vi "WPI_CameraBackground Loop.vi"(11 "CameraDevRef":T1) -> ()   [LabVIEW 2015]
doc: "This VI acquires the image buffer from the camera MJPG stream at the configured fps rate. It notifies any waiting VIs and allows them to pick up the latest image. This allows the camera and robot vision loop to run at different rates. The 1011, camera is far more efficient using MJPGs, and generally, this is probably the better choice for the camera loop.\n \nThis software is licensed. Open the labview\\readme\\WPI Robotics Library Open Source License.txt file for more information."
uses:
  <vilib>/Rock Robotics/WPI/Camera/WPI_CameraDevRef.ctl
  <vilib>/Rock Robotics/WPI/Camera/WPI_CameraSettings Operations.ctl
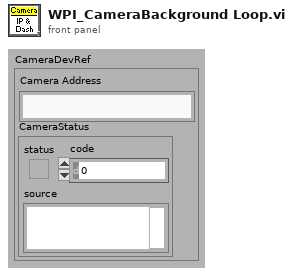
[diagram p1: front panel]
types:
  T1 = typedef "WPI_CameraDevRef.ctl" = cluster{"Camera Address":string, "CameraStatus":errorcluster}
  T2 = typedef "WPI_CameraSettings Operations.ctl" = enum16{"Udate FPS", "Update Compression", "Update Size", "Update White Balance", "Update Brightness", "Update Sharpness", "Update Exposure", "Update Exposure Value", "Update Color Level", "Update Exp Priority", "Update Color Enable", "Update JPG", "Update MJPG", "Read and Clear", "Read", "Init"}
  T3 = typedef "WPI_CameraSettings Control.ctl" = cluster{"FPS":i32, "Compression":i32, "Size":i32, "White Balance":i32, "Brightness":i32, "Sharpness":i32, "Exposure":i32, "Color Level":i32, "Exposure Priority":i32, "Color Enable":i32, "JPG Loop":i32, "MJPG Loop":i32, "Exposure Value":i32}
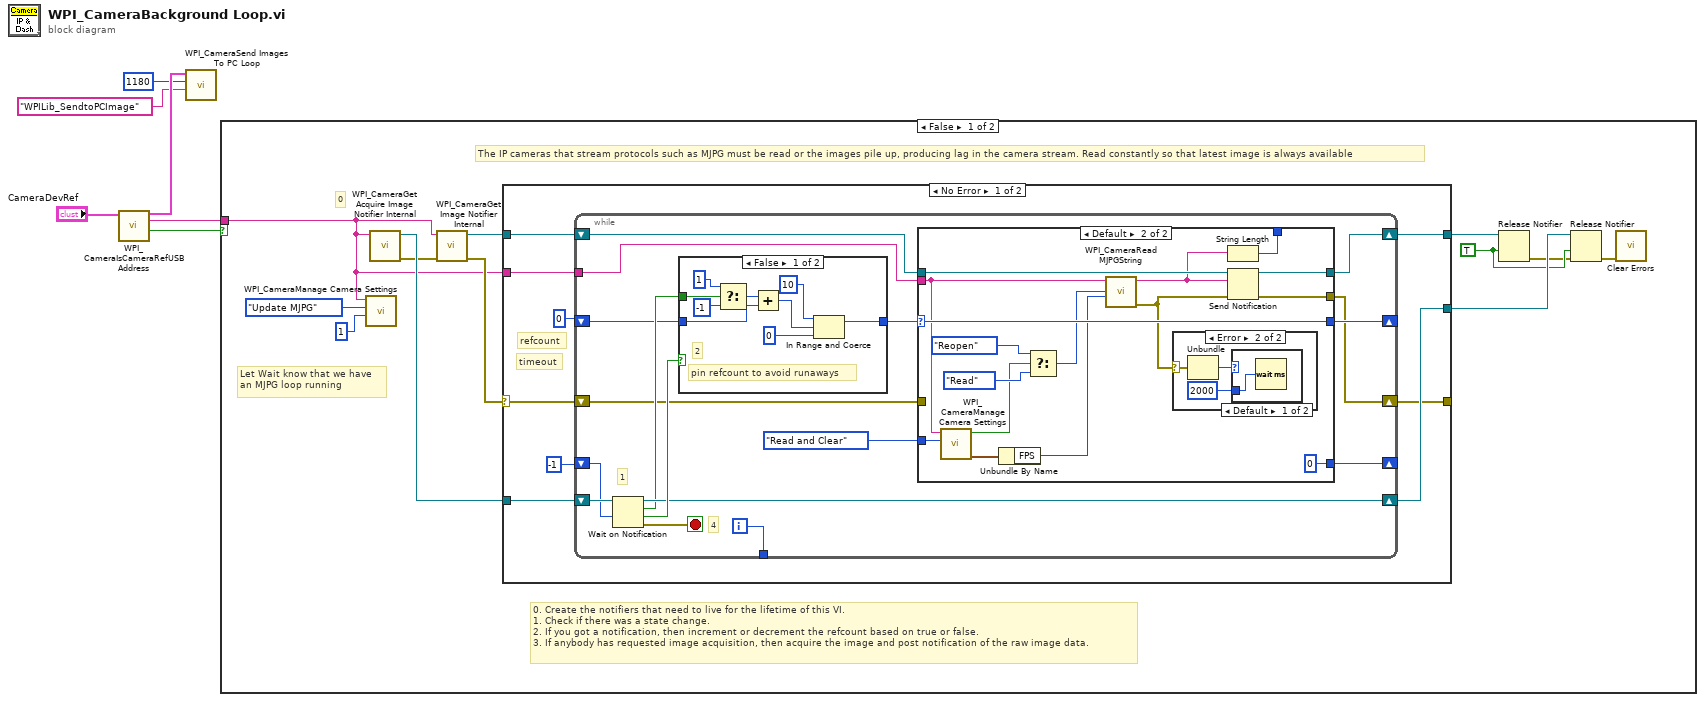
[diagram p0: block diagram]
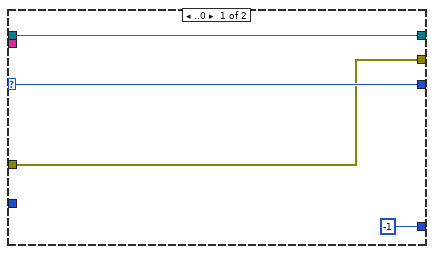
[diagram p2: hidden frame]
diagram:
  n1 = call <vilib>:"WPI_CameraIsCameraRefUSBAddress.vi"("CameraDevRef"="CameraDevRef") -> ("USB?"=w5:bool, "Camera Address Out"=w4:string, "CameraDevRef out"=w3:T1)  [unwired: 7 in, 1 out]
  n2 = call "WPI_CameraSend Images To PC Loop.vi"("String"="WPILib_SendtoPCImage", "port"=u16 1180, "CameraDevRef"=w3) -> ()  [unwired: 9 in]
  n3 = case shown="False" w5 {
    tunnel: w4 -> [w8 _]
    frame False {
      w15 = TRUE ("force destroy? (F)")
      # "The IP cameras that stream protocols such as MJPG must be read or the images pile up, producing lag in the camera stream. Read constantly so that latest image is always available"
      # "0. Create the notifiers that need to live for the lifetime of this VI. \n1. Check if there was a state change.\n2. If you got a notification, then increment or decrement the refcount based on true or false.\n3. If anybody has requested image acquisition, then acquire the image and post notification of the raw image data."
      # "Let Wait know that we have\nan MJPG loop running"
      # "0"
      n4 = call <vilib>:"WPI_CameraManage Camera Settings.vi"("Value"=1, "Operation"=WPI_CameraSettings_Operations."Update MJPG", "Camera IP"=w8) -> ()  [unwired: 7 in, 2 out]
      n5 = call <vilib>:"WPI_CameraGet Acquire Image Notifier Internal.vi"("Camera Address"=w8) -> ("error out"=w12:errorcluster, "Acquire Image Notifier"=w13:refnum<notifier>)  [unwired: 1 in, 8 out]
      n6 = call <vilib>:"WPI_CameraGet Image Notifier Internal.vi"("error in (no error)"=w12, "Camera Address"=w8) -> ("error out"=w14:errorcluster, "Image Notifier"=w16:refnum<notifier>)  [unwired: 8 out]
      n7 = case shown="No Error" w14 {
        selector: w14 -> [w20 w81]
        tunnel: w8 -> [w27 _]
        tunnel: w13 -> [w26 w79]
        tunnel: w16 -> [w24 w80]
        tunnel: [w22 w80] -> w18
        tunnel: [w21 w79] -> w17
        tunnel: [w19 w81] -> _
        frame No Error {
          # "timeout"
          # "refcount"
          n8 = while {
            shift-right: [w42] -> w21
            shift-left: w26 -> [w44]
            tunnel: w27 -> [w39]
            shift-right: [w31] -> _
            shift-left: 0 -> [w40]
            shift-right: [w37] -> w22
            shift-left: w24 -> [w38]
            shift-right: [w35] -> _
            shift-left: -1 -> [w36]
            shift-right: [w30] -> w19
            shift-left: w20 -> [w33]
            tunnel: [w28] -> _
            i -> [w28]
            stop <- w34 stop-if-true
            # "4"
            # "1"
            n9 = Wait on Notification(notifier=w44, timeout in ms (-1)=w36) -> (notifier out=w42:refnum<notifier>, notification=w41:bool, timed out?=w43:bool, error out=w34:errorcluster)  [unwired: 1 in, 1 out]
            n10 = case shown="False" w43 {
              tunnel: w41 -> [w77 _]
              tunnel: w40 -> [w73 w78]
              tunnel: [w69 w78] -> w32
              frame False {
                # "pin refcount to avoid runaways"
                # "2"
                n11 = Select(t=1, s=w77, f=-1) -> (s? t:f=w74:i32)
                n12 = Add(x=w74, y=w73) -> (x+y=w70:i32)
                n13 = In Range and Coerce(upper limit=10, x=w70, lower limit=0) -> (coerced(x)=w69:i32)  [unwired: 1 out]
              }
              frame True {
              }
            }
            n14 = case shown="Default" w32 {
              selector: w32 -> [w47 w61]
              tunnel: w39 -> [_ w49]
              tunnel: w38 -> [w48 w64]
              tunnel: [w48 w63] -> w37
              tunnel: [-1 0] -> w35
              tunnel: w33 -> [w45 _]
              tunnel: [w47 w61] -> w31
              tunnel: [w45 w60] -> w30
              tunnel: [_ w54] -> _
              tunnel: WPI_CameraSettings_Operations."Read and Clear" ("Operation") -> [_ w50]
              frame ..0 {
              }
              frame Default {
                n15 = call <vilib>:"WPI_CameraManage Camera Settings.vi"("Operation"=w50, "Camera IP"=w49) -> ("Values"=w52:T3, "Changed"=w53:bool)  [unwired: 8 in]
                n16 = Unbundle By Name(w52) -> ("FPS"=w51:i32)
                n17 = Select(t=enum16{"Read", "Reopen", "Close"}."Reopen" ("Operation"), s=w53, f=enum16{"Read", "Reopen", "Close"}."Read" ("Operation")) -> (s? t:f=w56:enum16{"Read", "Reopen", "Close"})
                n18 = call <vilib>:"WPI_CameraRead MJPGString.vi"("fps"=w51, "Operation"=w56, "address"=w49) -> ("error out"=w59:errorcluster, "Raw Image Data"=w55:string)  [unwired: 7 in]
                n19 = case shown="Error" w59 {
                  selector: w59 -> [_ w67]
                  frame No Error {
                  }
                  frame Error {
                    n20 = Unbundle(w67) -> ("code"=w66:i32)  [unwired: 2 out]
                    n21 = case shown="Default" w66 {
                      tunnel: u32 2000 ("milliseconds to wait") -> [w68 _]
                      frame Default {
                        n22 = Wait (ms)(milliseconds to wait=w68) -> ()  [unwired: 1 out]
                      }
                      frame 56 {
                      }
                    }
                  }
                }
                n23 = String Length(string=w55) -> (length=w54:i32)
                n24 = Send Notification(notification=w55, notifier=w64, error in (no error)=w59) -> (notifier out=w63:refnum<notifier>, error out=w60:errorcluster)
              }
            }
          }
        }
        frame Error {
        }
      }
      n25 = Release Notifier(notifier=w18, force destroy? (F)=w15) -> (error out=w11:errorcluster)  [unwired: 1 in, 2 out]
      n26 = Release Notifier(notifier=w17, force destroy? (F)=w15, error in (no error)=w11) -> (error out=w7:errorcluster)  [unwired: 2 out]
      n27 = call <vilib>:"Clear Errors.vi"("error in (no error)"=w7) -> ()  [unwired: 1 in, 6 out]
    }
    frame True {
      # "The USB cameras may need to be forwarded over ethernet. Read, compress, and send to the Dashbd."
    }
  }
